vi "GetReferenceState.vi"(9 "CThread Reference":refnum<vi>, 19 "error in (no error)":errorcluster) -> (8 "VI Name":string, 10 "VI Path":path, 12 "Clone":i16, 14 "Encoded Name":u32, 18 "error out":errorcluster)   [LabVIEW 2012, in "CThread.lvlib"]
uses:
  CThread.lvlib
  State.ctl
  CThread VI Reference.xnode
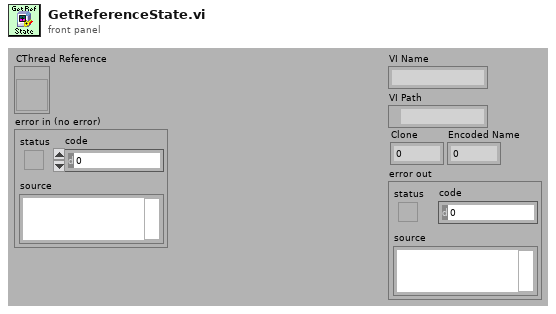
[diagram p1: front panel]
types:
  T1 = typedef "CThread.lvlib/CThread VI Reference.xnode/State.ctl" = cluster{"VI Name":string, "VI Path":path, "Clone":i16, "Encoded Name":u32}
  T2 = cluster{"Library Version":cluster{"Major":u16, "Minor":u16, "Fix":u16, "Build":u16}, "State":variant}
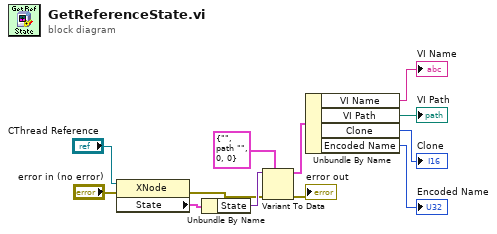
[diagram p0: block diagram]
diagram:
  n1 = property class="XNode"(reference="CThread Reference", error in="error in (no error)") -> (error out=w3:errorcluster, "State"=w12:T2)  [unwired: 1 out]
  n2 = Unbundle By Name(w12) -> ("State"=w11:variant)
  n3 = Variant To Data(error in=w3, type=T1 {"VI Name"="", "VI Path"=path "", "Clone"=0, "Encoded Name"=0} ("State"), Variant=w11) -> (data=w9:T1, error out=→"error out":errorcluster)
  n4 = Unbundle By Name(w9) -> ("VI Name"=→"VI Name":string, "VI Path"=→"VI Path":path, "Clone"=→"Clone":i16, "Encoded Name"=→"Encoded Name":u32)
